vi "remove no error default.vi"() -> ()   [LabVIEW 2013]
uses:
  <vilib>/Utility/VariantDataType/VariantType.lvlib
panel:
  out "errors":errorcluster[](array[cluster])
  in  "Folder Path":path
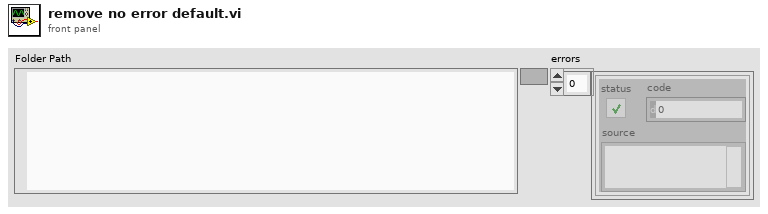
[diagram p1: front panel]
types:
  T1 = typedef "VariantType.lvlib/Type.ctl" = enum8{"Invalid Type", "Void", "I8", "I16", "I32", "I64", "U8", "U16", "U32", "U64", "Single Float", "Double Float", "Extended Float", "Single Complex", "Double Complex", "Extended Complex", "Enum U8", "Enum U16", "Enum U32", "Enum U64", "Single Float With Unit", "Double Float With Unit", "Extended Float With Unit", "Single Complex with Unit", "Double Complex with Unit", "Extended Complex with Unit", "Boolean", "String", "Path", "Picture", "Tag", "Array", "Cluster", "Variant", "LV Variant", "Waveform", "Timestamp", "Digital Waveform", "Digital Data", "ExpressData", "Refnum", "External Data", "VI", "Poly VI", "LabVIEW Class Instance", "Fixed Point"}
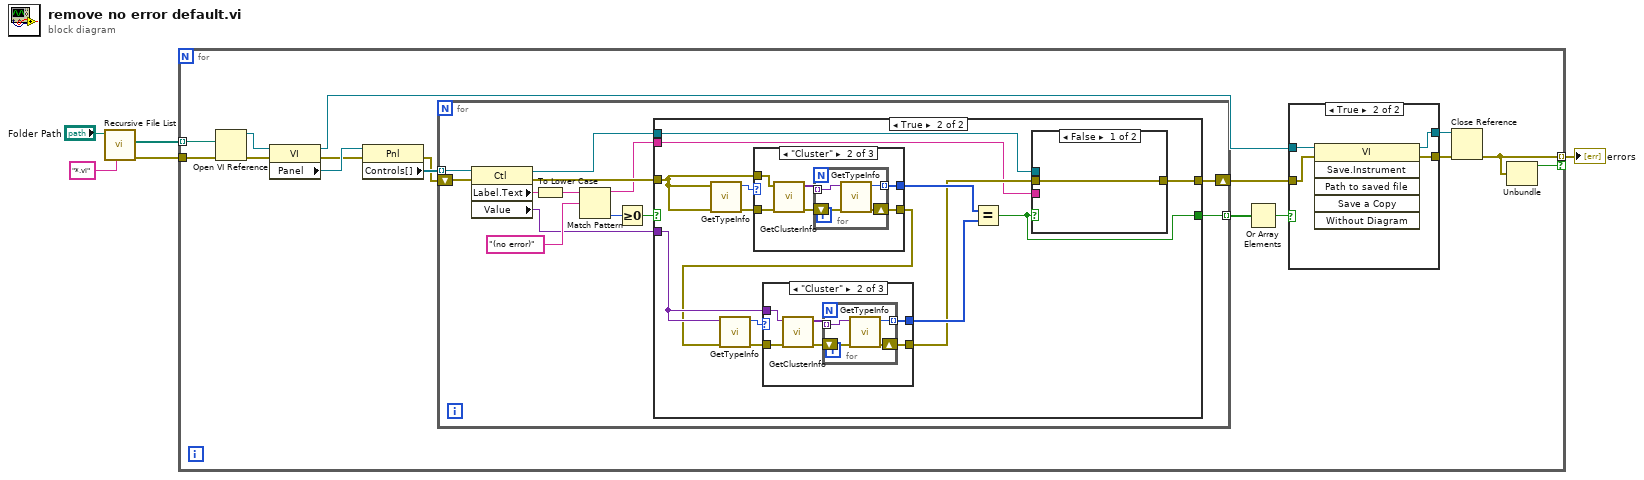
[diagram p0: block diagram]
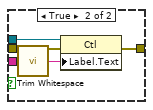
[diagram p3: hidden frame]
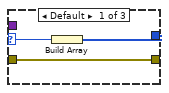
[diagram p4: hidden frame]
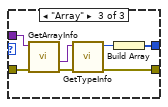
[diagram p5: hidden frame]
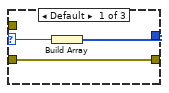
[diagram p6: hidden frame]
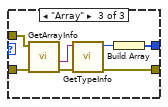
[diagram p7: hidden frame]
diagram:
  n1 = call <vilib>:"Recursive File List.vi"("pattern"="*.vi", "Folder Path"="Folder Path") -> ("error out"=w2:errorcluster, "All Files in Dir"=w3:path[])  [unwired: 5 in, 3 out]
  n2 = for {
    tunnel: w3 -> [w20] mode=indexing
    tunnel: w2 -> [w21]
    tunnel: [w19] -> w1 mode=indexing if=w18
    n3 = Open VI Reference(vi path=w20, error in (no error)=w21) -> (vi reference=w16:refnum<vi>, error out=w17:errorcluster)  [unwired: 4 in]
    n4 = property class="VI"(reference=w16, error in=w17) -> (reference out=w12:refnum<vi>, error out=w14:errorcluster, "Panel"=w15:refnum<vi>)
    n5 = property class="Pnl"(reference=w15, error in=w14) -> (error out=w9:errorcluster, "Controls[]"=w10:refnum<vi>[])  [unwired: 1 out]
    n6 = for {
      tunnel: w10 -> [w34] mode=indexing
      shift-right: [w24] -> w6
      shift-left: w9 -> [w33]
      tunnel: [w26] -> w7 mode=indexing
      n7 = property class="Ctl"(reference=w34, error in=w33) -> (reference out=w23:refnum<vi>, error out=w25:errorcluster, "Label.Text"=w32:string, "Value"=w27:variant)
      n8 = To Lower Case(string=w32) -> (all lower case string=w31:string)
      n9 = Match Pattern(string=w31, regular expression="(no error)") -> (before substring=w22:string, offset past match=w29:i32)  [unwired: 1 in, 2 out]
      n10 = Greater Or Equal To 0?(x=w29) -> (x >= 0?=w28:bool)
      n11 = case shown="True" w28 {
        selector: w28 -> [w36 _]
        tunnel: w27 -> [_ w45]
        tunnel: [w36 w37] -> w26
        tunnel: w25 -> [w35 w48]
        tunnel: [w35 w40] -> w24
        tunnel: w23 -> [_ w39]
        tunnel: w22 -> [_ w38]
        frame False {
        }
        frame True {
          n12 = call <vilib>:"GetTypeInfo.vi"("error in (no error)"=w48, "Variant"=w48) -> ("error out"=w49:errorcluster, "Type Enum"=w50:T1)  [unwired: 5 in, 3 out]
          n13 = case shown="\"Cluster\"" w50 {
            selector: w50 -> [w79 _ _]
            tunnel: w48 -> [_ w85 w96]
            tunnel: [w78 w83 w93] -> w43
            tunnel: w49 -> [w77 w82 w91]
            tunnel: [w77 w80 w90] -> w44
            frame Default {
              n14 = Build Array(w79) -> (w78:T1[])
            }
            frame "Cluster" {
              n15 = call <vilib>:"GetClusterInfo.vi"("error in (no error)"=w82, "Variant"=w85) -> ("error out"=w81:errorcluster, "Cluster Elements"=w84:variant[])  [unwired: 8 in]
              n16 = for {
                tunnel: w84 -> [w89] mode=indexing
                tunnel: [w88] -> w83 mode=indexing
                shift-right: [w87] -> w80
                shift-left: w81 -> [w86]
                n17 = call <vilib>:"GetTypeInfo.vi"("error in (no error)"=w86, "Variant"=w89) -> ("error out"=w87:errorcluster, "Type Enum"=w88:T1)  [unwired: 5 in, 3 out]
              }
            }
            frame "Array" {
              n18 = call <vilib>:"GetArrayInfo.vi"("error in (no error)"=w91, "Variant"=w96) -> ("error out"=w92:errorcluster, "ArrayElement"=w95:variant)  [unwired: 6 in, 2 out]
              n19 = call <vilib>:"GetTypeInfo.vi"("error in (no error)"=w92, "Variant"=w95) -> ("error out"=w90:errorcluster, "Type Enum"=w94:T1)  [unwired: 5 in, 3 out]
              n20 = Build Array(w94) -> (w93:T1[])
            }
          }
          n21 = call <vilib>:"GetTypeInfo.vi"("error in (no error)"=w44, "Variant"=w45) -> ("error out"=w47:errorcluster, "Type Enum"=w46:T1)  [unwired: 5 in, 3 out]
          n22 = case shown="\"Cluster\"" w46 {
            selector: w46 -> [w59 _ _]
            tunnel: w45 -> [_ w65 w76]
            tunnel: [w58 w63 w73] -> w42
            tunnel: w47 -> [w57 w62 w71]
            tunnel: [w57 w60 w70] -> w41
            frame Default {
              n23 = Build Array(w59) -> (w58:T1[])
            }
            frame "Cluster" {
              n24 = call <vilib>:"GetClusterInfo.vi"("error in (no error)"=w62, "Variant"=w65) -> ("error out"=w61:errorcluster, "Cluster Elements"=w64:variant[])  [unwired: 8 in]
              n25 = for {
                tunnel: w64 -> [w69] mode=indexing
                tunnel: [w68] -> w63 mode=indexing
                shift-right: [w67] -> w60
                shift-left: w61 -> [w66]
                n26 = call <vilib>:"GetTypeInfo.vi"("error in (no error)"=w66, "Variant"=w69) -> ("error out"=w67:errorcluster, "Type Enum"=w68:T1)  [unwired: 5 in, 3 out]
              }
            }
            frame "Array" {
              n27 = call <vilib>:"GetArrayInfo.vi"("error in (no error)"=w71, "Variant"=w76) -> ("error out"=w72:errorcluster, "ArrayElement"=w75:variant)  [unwired: 6 in, 2 out]
              n28 = call <vilib>:"GetTypeInfo.vi"("error in (no error)"=w72, "Variant"=w75) -> ("error out"=w70:errorcluster, "Type Enum"=w74:T1)  [unwired: 5 in, 3 out]
              n29 = Build Array(w74) -> (w73:T1[])
            }
          }
          n30 = Equal?(x=w43, y=w42) -> (x = y?=w37:bool)
          n31 = case shown="False" w37 {
            tunnel: w41 -> [w51 w56]
            tunnel: [w51 w55] -> w40
            tunnel: w39 -> [_ w54]
            tunnel: w38 -> [_ w52]
            frame False {
            }
            frame True {
              n32 = call <vilib>:"Trim Whitespace.vi"("string"=w52) -> ("trimmed string"=w53:string)  [unwired: 1 in]
              n33 = property class="Ctl"(reference=w54, error in=w56, "Label.Text"=w53) -> (error out=w55:errorcluster)  [unwired: 1 out]
            }
          }
        }
      }
    }
    n34 = Or Array Elements(Boolean array=w7) -> (logical OR=w8:bool)
    n35 = case shown="True" w8 {
      tunnel: [w97 w102] -> w13
      tunnel: w12 -> [w98 w101]
      tunnel: [w98 w100] -> w11
      tunnel: w6 -> [w97 w99]
      frame False {
      }
      frame True {
        n36 = invoke class="VI" method="Save.Instrument"(reference=w101, error in=w99) -> (reference out=w100:refnum<vi>, error out=w102:errorcluster)  [unwired: 4 in, 4 out]
      }
    }
    n37 = Close Reference(reference=w11, error in (no error)=w13) -> (error out=w19:errorcluster)
    n38 = Unbundle(w19) -> ("status"=w18:bool)  [unwired: 2 out]
  }
  "errors" <- w1
